vi "Initialize.vi"(8 "error in (no error)":errorcluster, 10 "DAQ Class.lvclass":refnum<class "DAQ Class.lvclass">, 11 "Processing in":refnum<class "Processing.lvclass">) -> (0 "error out":errorcluster, 3 "Processing out":refnum<class "Processing.lvclass">)   [LabVIEW 2015, in "Processing.lvclass"]
uses:
  Processing.lvclass
  DAQ/DAQ Class.lvclass
  Galvo/Galvo.lvclass
panel:
  in  "Galvo.lvclass":refnum<class "Galvo.lvclass">
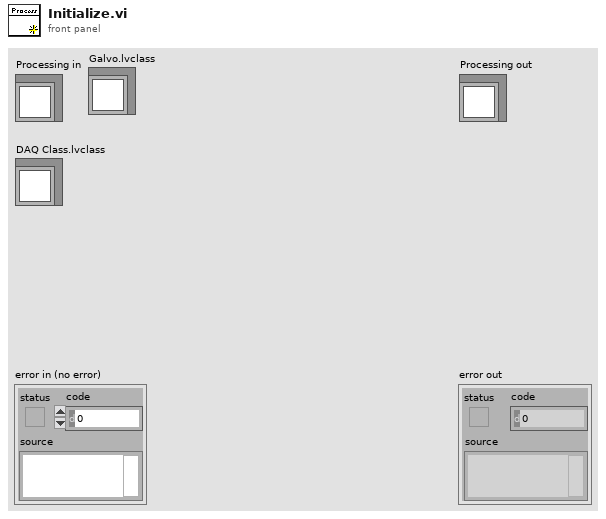
[diagram p1: front panel]
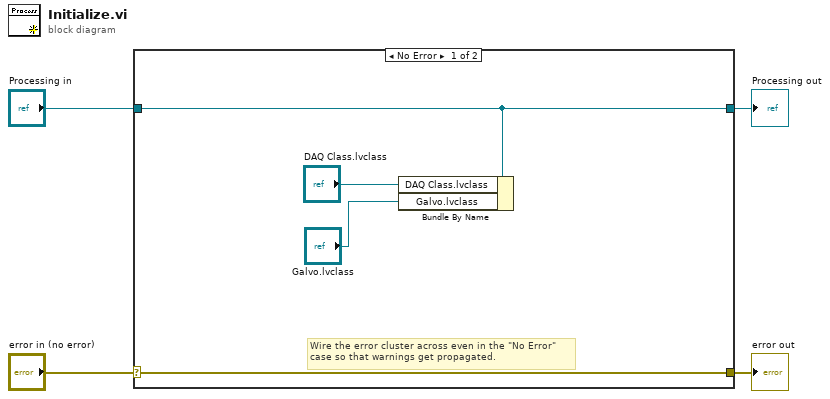
[diagram p0: block diagram]
diagram:
  n1 = case shown="No Error" "error in (no error)" {
    selector: "error in (no error)" -> [w8 w10]
    tunnel: [w8 w10] -> w3
    tunnel: [w7 w9] -> w1
    tunnel: "Processing in" -> [w7 w9]
    frame No Error {
      # "Wire the error cluster across even in the \"No Error\"\ncase so that warnings get propagated."
      n2 = Bundle By Name(cluster=w7, "DAQ Class.lvclass"="DAQ Class.lvclass", "Galvo.lvclass"="Galvo.lvclass") -> ()  [unwired: 1 out]
    }
    frame Error {
    }
  }
  "error out" <- w3
  "Processing out" <- w1
